vi "rs3 get failed args.vi"(8 "error in (no error)":errorcluster, 11 "error in":u64) -> (0 "error out":errorcluster, 2 "error out":u64, 3 "Failed args":string)   [LabVIEW 2017, in "libRealSense3.lvlib"]
doc: "const char * rs_get_failed_args (const rs_error * error);"
uses:
  libRealSense3.lvlib
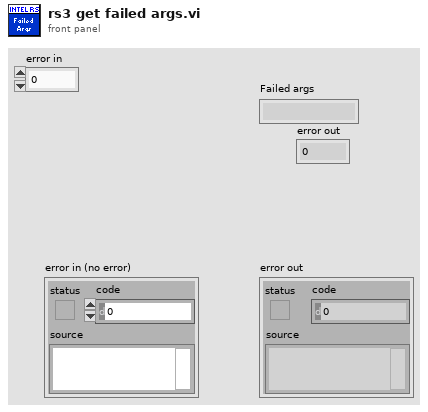
[diagram p1: front panel]
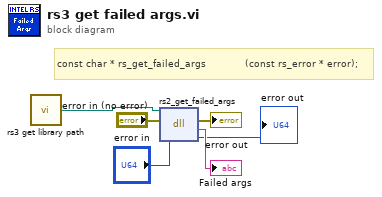
[diagram p0: block diagram]
diagram:
  # "const char * rs_get_failed_args             (const rs_error * error);"
  n1 = call "rs3 get library path.vi"() -> ("Realsense 2 Library Path"=w1:path)
  n2 = dll-call lib="C:/Users/agrunnet/Documents/libRealSense6/realsense2.dll" fn="rs2_get_failed_args"(path in=w1, error in="error in (no error)", "error"="error in") -> (error out=→"error out":errorcluster, "return type"=→"Failed args":string, "error"=→"error out":u64)  [unwired: 1 in, 1 out]
